vi "choose_settings_dialog.vi"(8 "error in (no error)":errorcluster, 10 "settings in":T1, 11 "GenericPlugin in":refnum<class "GenericComponent.lvclass">) -> (0 "error out":errorcluster, 1 "cancelled?":bool, 2 "settings out":T1, 3 "GenericPlugin out":refnum<class "GenericComponent.lvclass">)   [LabVIEW 2010, in "GenericComponent.lvclass"]
uses:
  GenericComponent.lvclass
  clusters/settings_specification_cluster.ctl
  clusters/plugin_specification.ctl
panel:
  in  "Settings file":string(combo)
  in  "Label":string
  in  "cancel button":bool
  in  "ok button":bool
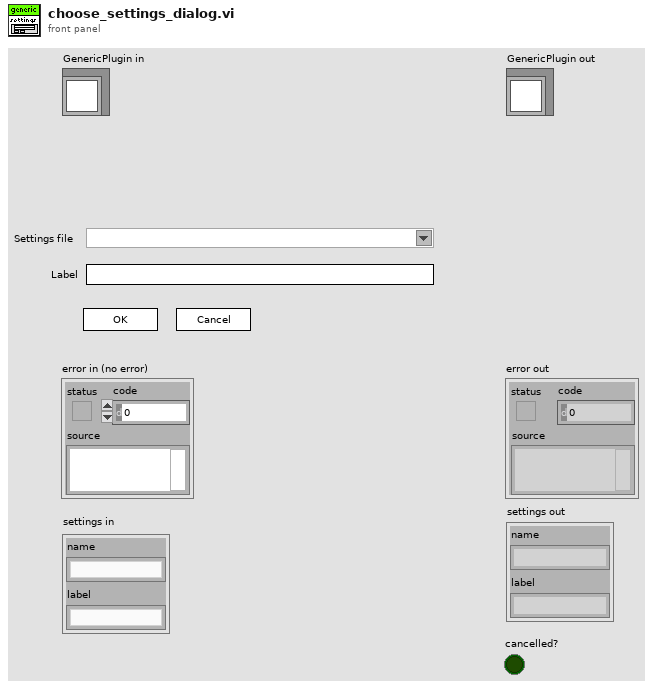
[diagram p1: front panel]
types:
  T1 = typedef "settings_specification_cluster.ctl" = cluster{"name":string, "label":string}
  T2 = typedef "plugin_specification.ctl" = cluster{"class path":string, "configuration":string, "label":string, "settings name":string}
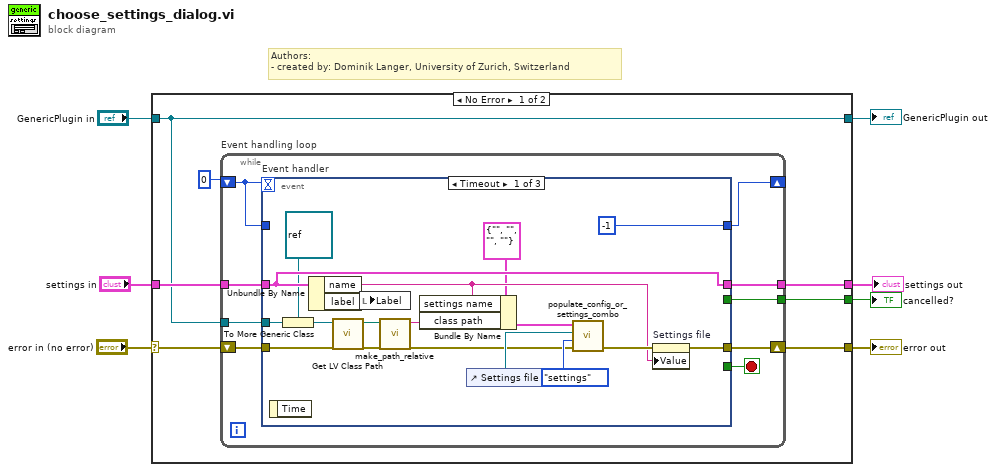
[diagram p0: block diagram]
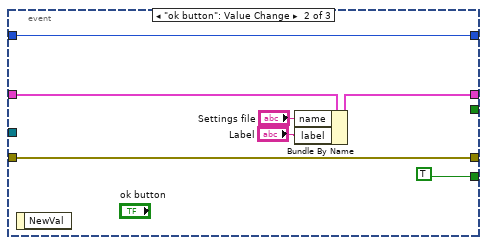
[diagram p2: hidden frame]
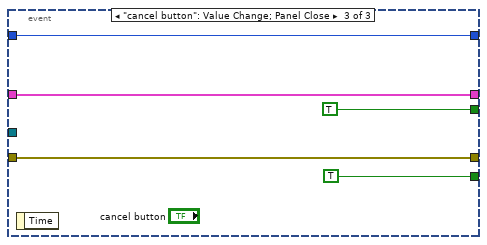
[diagram p3: hidden frame]
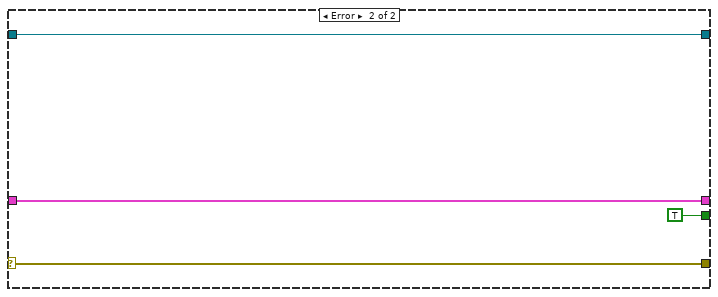
[diagram p4: hidden frame]
diagram:
  # "Authors: \n- created by: Dominik Langer, University of Zurich, Switzerland"
  n1 = case shown="No Error" "error in (no error)" {
    selector: "error in (no error)" -> [w9 w57]
    tunnel: [w14 w57] -> w6
    tunnel: [w12 TRUE] -> w7
    tunnel: [w8 w55] -> w3
    tunnel: "GenericPlugin in" -> [w8 w55]
    tunnel: "settings in" -> [w11 w54]
    tunnel: [w10 w54] -> w1
    frame No Error {
      n2 = while "Event handling loop" {
        shift-right: [w22] -> w14
        shift-left: w9 -> [w23]
        shift-right: [w20] -> _
        shift-left: 0 -> [w21]
        tunnel: [w18] -> w12
        tunnel: w11 -> [w17]
        tunnel: [w16] -> w10
        tunnel: w8 -> [w15]
        stop <- w19 stop-if-true
        n3 = event "Event handler" shown="[0] Timeout" {
          selector: _ -> [_ _ _]
          dyn-events: _ -> [_ _ _]
          timeout: w21 -> [_ _ _]
          tunnel: [w37 w48 w53] -> w22
          tunnel: w23 -> [w34 w48 w53]
          tunnel: [-1 w47 w52] -> w20
          tunnel: w21 -> [_ w47 w52]
          tunnel: [_ TRUE TRUE] -> w19
          tunnel: [_ _ TRUE] -> w18
          tunnel: w17 -> [w36 w45 w49]
          tunnel: [w36 w44 w49] -> w16
          tunnel: w15 -> [w32 _ _]
          event Timeout {
            n4 = event-data() -> ()  [unwired: 1 in, 1 out]
            n5 = To More Generic Class(target class=refnum<class> refnum ("LabVIEW Object"), reference=w32) -> (generic class reference=w31:refnum<class>)
            n6 = Unbundle By Name(w36) -> ("name"=w30:string, "label"=w35:string)
            n7 = call <vilib>:"Get LV Class Path.vi"("error in (no error)"=w34, "object"=w31) -> ("error out"=w28:errorcluster, "class path"=w26:path)  [unwired: 8 in]
            n8 = local write "Label"(w35) -> ()
            n9 = call "make_path_relative.vi"("error in (no error)"=w28, "absolute path"=w26) -> ("error out"=w27:errorcluster, "relative path"=w25:string)  [unwired: 8 in]
            n10 = Bundle By Name(cluster=T2 {"class path"="", "configuration"="", "label"="", "settings name"=""} ("plug-in specification"), "settings name"=w30, "class path"=w25) -> (w24:T2)
            n11 = control-ref of="Settings file"() -> (w39:refnum<vi>)
            n12 = call "populate_config_or_settings_combo.vi"("error in (no error)"=w27, "type"=enum16{"configuration", "settings"}."settings", "combo-box reference"=w39, "plug-in specification"=w24) -> ("error out"=w38:errorcluster)  [unwired: 7 in]
            n13 = property on="Settings file" class="CmbBox"(error in=w38, "Value"=w30) -> (error out=w37:errorcluster)  [unwired: 1 in, 1 out]
          }
          event "ok button": Value Change {
            n14 = event-data() -> ()  [unwired: 1 in, 1 out]
            n15 = Bundle By Name(cluster=w45, "name"="Settings file", "label"="Label") -> (w44:T1)
          }
          event "cancel button": Value Change; Panel Close {
            n16 = event-data() -> ()  [unwired: 1 in, 1 out]
          }
        }
      }
    }
    frame Error {
    }
  }
  "error out" <- w6
  "GenericPlugin out" <- w3
  "cancelled?" <- w7
  "settings out" <- w1
